vi "DEV Select bad.vi"(8 "error in (no error)":errorcluster, 9 "String Values":string[](array[string]), 10 "Columns":string[](array[string]), 11 "Database":string) -> (0 "error out":errorcluster, 2 "Output Data":string[][](array[string]), 3 "Query [Debug]":string)   [LabVIEW 2018, in "Database.lvlib"]
uses:
  Database.lvlib
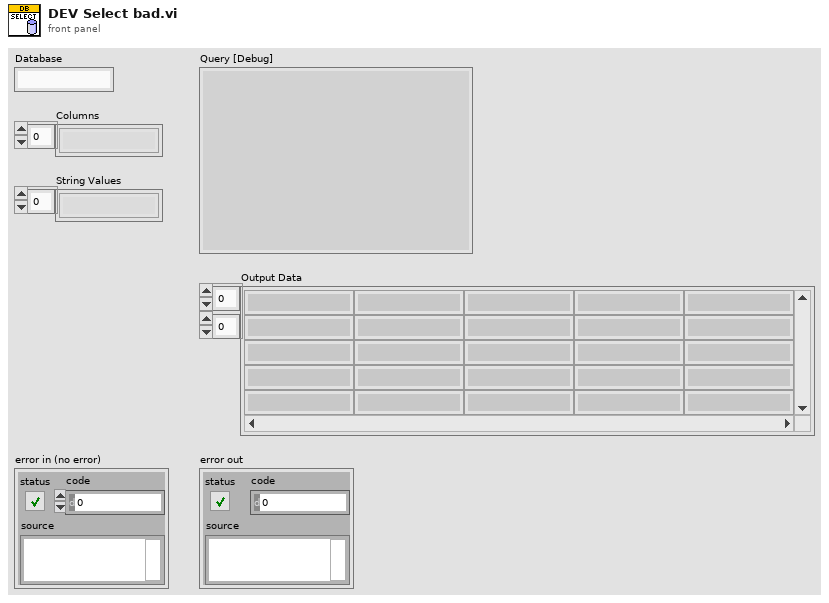
[diagram p1: front panel]
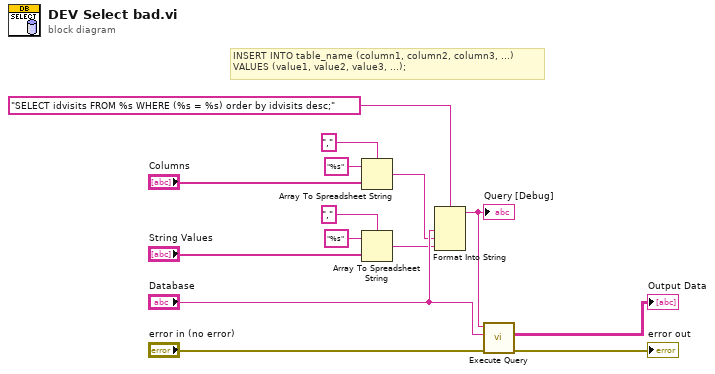
[diagram p0: block diagram]
diagram:
  # "INSERT INTO table_name (column1, column2, column3, ...)\nVALUES (value1, value2, value3, ...);"
  n1 = Array To Spreadsheet String(delimiter (Tab)=",", array="Columns", 3:"%s" ("format string")) -> (spreadsheet string=w8:string)
  n2 = Array To Spreadsheet String(delimiter (Tab)=",", array="String Values", 3:"%s" ("format string")) -> (spreadsheet string=w9:string)
  n3 = Format Into String(format string="SELECT idvisits FROM %s WHERE (%s = %s) order by idvisits desc;", "Database", w8, w9) -> (resulting string=w11:string)  [unwired: 2 in, 1 out]
  "Query [Debug]" <- w11
  n4 = call "Execute Query.vi"("Error In"="error in (no error)", "Table"="Database", "Query"=w11) -> ("Error Out"=→"error out":errorcluster, "Output Data"=→"Output Data":string[][])  [unwired: 6 in, 1 out]
